vi "Test Modbus.vi"() -> ()   [LabVIEW 2020]
uses:
  <vilib>/NI/Modbus Library/API/Modbus API.lvclass/Modbus API.ctl
  <vilib>/NI/Modbus Library/Transmission Data Unit/Transmission Data Unit.lvclass/Transmission Data Unit.ctl
  <vilib>/NI/Modbus Library/Transmission Data Unit/Write Unit ID.vi
  <vilib>/NI/Modbus Library/API/Read Transmission Data Unit.vi
  <vilib>/NI/Modbus Library/API/Write Transmission Data Unit.vi
  <vilib>/NI/Modbus Library/API/Master/Modbus Master.lvclass
  C:/Program Files (x86)/National Instruments/LabVIEW 2020/vi.lib/NI/Modbus Library/API/Modbus API.lvclass
  <vilib>/NI/Modbus Library/API/Wrapper/Create TCP Master.vi
  <vilib>/NI/Modbus Library/API/Wrapper/API Main.lvlib
panel:
  out "Array 2":dbl[](array[numeric])
  in  "Btn_Set Unit ID":bool
  in  "unit ID":u8
  in  "Array":T1(array[cluster])
  in  "stop":bool
  in  "port (502)":u16=502
  in  "address":string
  in  "Btn_Connect":bool
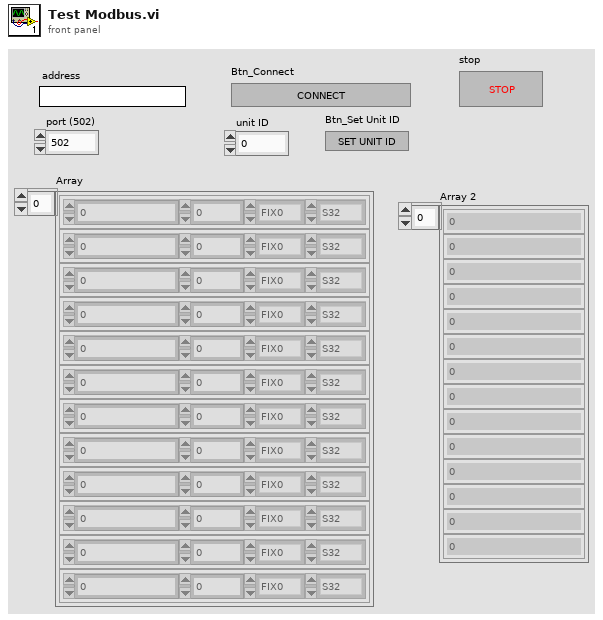
[diagram p1: front panel]
types:
  T1 = cluster{"starting address":u16, "number of inputs":u16, "Data Format":enum16{"FIX0", "FIX1", "FIX2", "FIX3", "FIX4", "FIX5", "FIX6"}, "Data Type":enum16{"S32", "U32"}}[]
  T2 = enum16{"FIX0", "FIX1", "FIX2", "FIX3", "FIX4", "FIX5", "FIX6"}
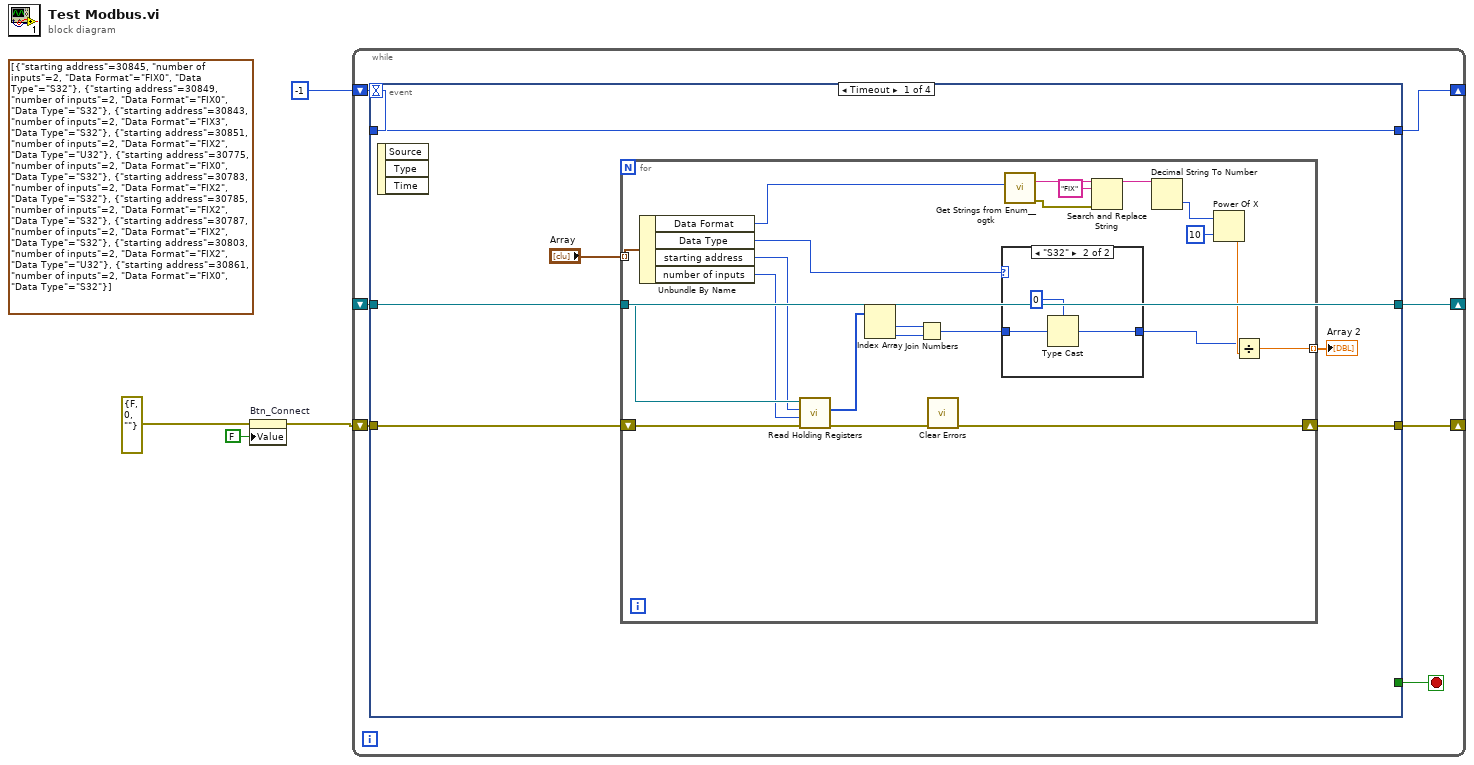
[diagram p0: block diagram]
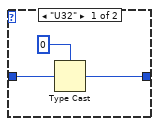
[diagram p2: hidden frame]
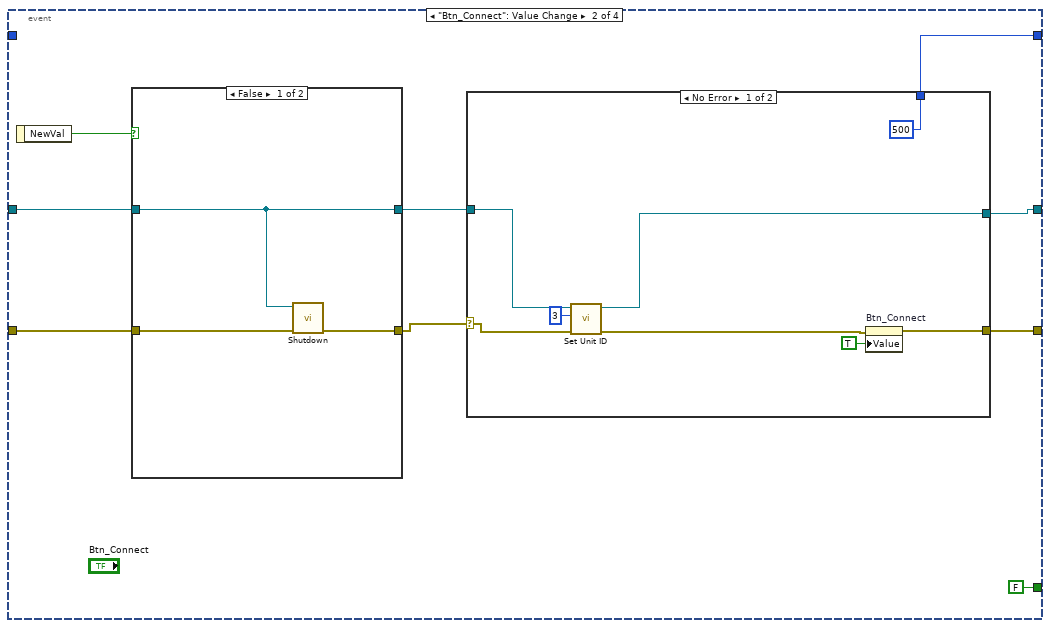
[diagram p3: hidden frame]
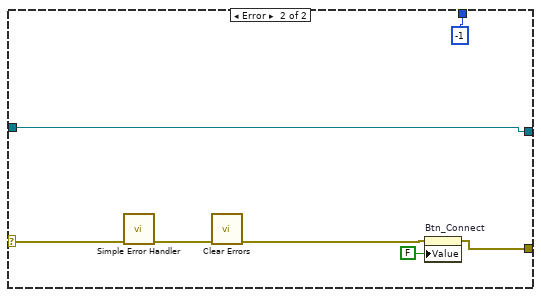
[diagram p4: hidden frame]
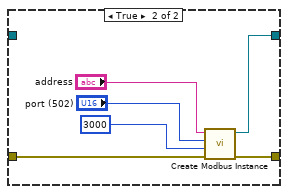
[diagram p5: hidden frame]
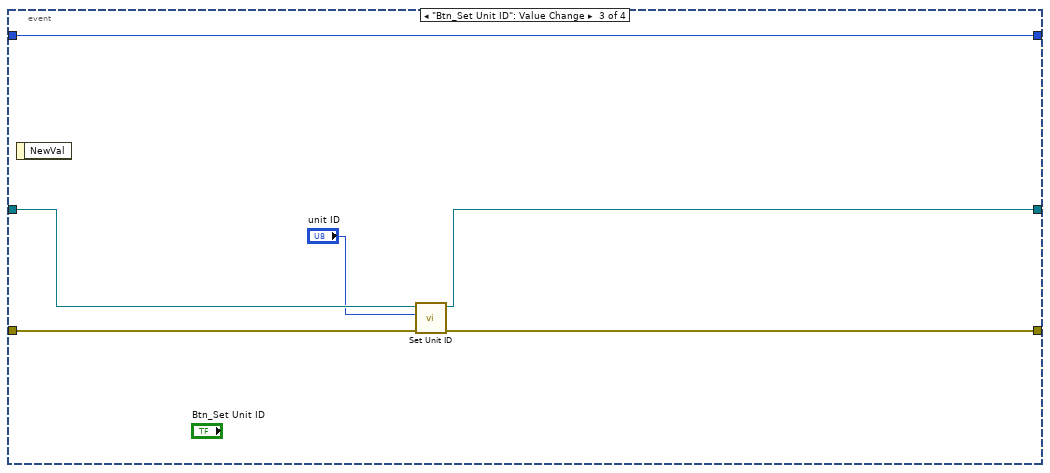
[diagram p6: hidden frame]
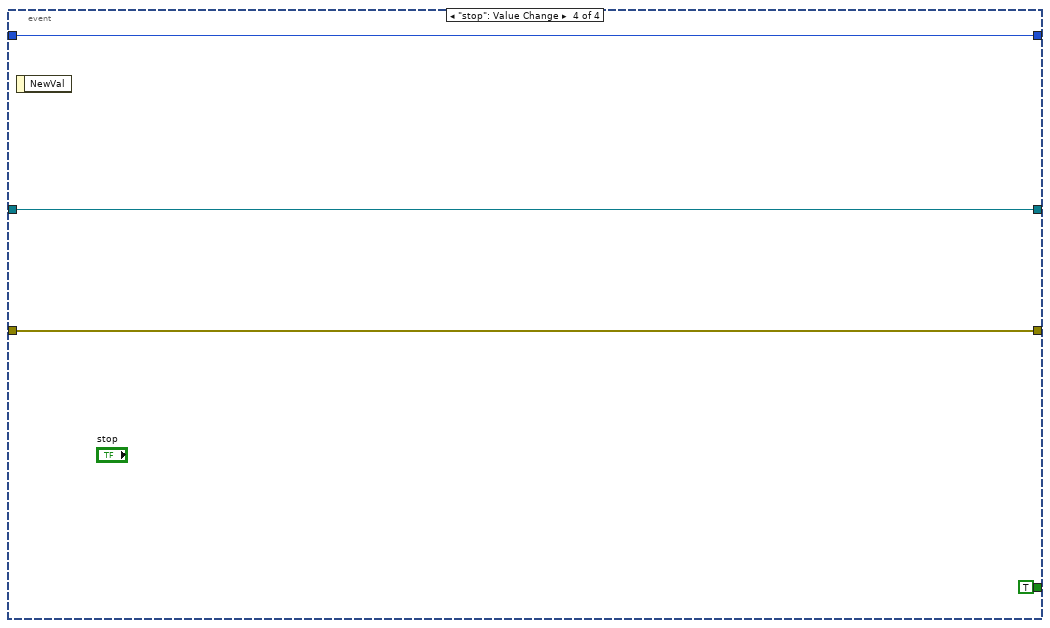
[diagram p7: hidden frame]
diagram:
  (unwired) T1 [{"starting address"=30845, "number of inputs"=2, "Data Format"=enum."FIX0", "Data Type"=enum."S32"}, {"starting address"=30849, "number of inputs"=2, "Data Format"=enum."FIX0", "Data Type"=enum."S32"}, {"starting address"=30843, "number of inputs"=2, "Data Format"=enum."FIX3", "Data Type"=enum."S32"}, {"starting address"=30851, "number of inputs"=2, "Data Format"=enum."FIX2", "Data Type"=enum."U32"}, {"starting address"=30775, "number of inputs"=2, "Data Format"=enum."FIX0", "Data Type"=enum."S32"}, {"starting address"=30783, "number of inputs"=2, "Data Format"=enum."FIX2", "Data Type"=enum."S32"}, {"starting address"=30785, "number of inputs"=2, "Data Format"=enum."FIX2", "Data Type"=enum."S32"}, {"starting address"=30787, "number of inputs"=2, "Data Format"=enum."FIX2", "Data Type"=enum."S32"}, {"starting address"=30803, "number of inputs"=2, "Data Format"=enum."FIX2", "Data Type"=enum."U32"}, {"starting address"=30861, "number of inputs"=2, "Data Format"=enum."FIX0", "Data Type"=enum."S32"}] ("Array")
  n1 = property on="Btn_Connect" class="Bool (strict)"(error in=errorcluster {"status"=FALSE, "code"=0, "source"=""} ("error out"), "Value"=FALSE ("Btn_Connect")) -> (error out=w3:errorcluster)  [unwired: 1 in, 1 out]
  n2 = while {
    shift-right: [w5] -> _
    shift-left: w3 -> [w11]
    shift-right: [w10] -> _
    shift-left: _ -> [w9]
    shift-right: [w6] -> _
    shift-left: -1 -> [w7]
    stop <- w8 stop-if-true
    n3 = event shown="[0] Timeout" {
      selector: _ -> [_ _ _ _]
      dyn-events: _ -> [_ _ _ _]
      timeout: w7 -> [_ _ _ _]
      tunnel: [w15 w50 w83 w87] -> w5
      tunnel: w11 -> [w16 w53 w84 w87]
      tunnel: [w14 w47 w81 w86] -> w10
      tunnel: w9 -> [w14 w52 w82 w86]
      tunnel: [_ FALSE _ TRUE] -> w8
      tunnel: w7 -> [w17 _ w79 w85]
      tunnel: [w17 w49 w79 w85] -> w6
      event Timeout {
        n4 = event-data() -> ()  [unwired: 1 in, 3 out]
        n5 = for {
          tunnel: w14 -> [w37]
          shift-right: [w29] -> w15
          shift-left: w16 -> [w39]
          tunnel: "Array" -> [w36] mode=indexing
          tunnel: [w30] -> w12 mode=indexing
          n6 = Unbundle By Name(w36) -> ("Data Format"=w21:T2, "Data Type"=w20:enum16{"S32", "U32"}, "starting address"=w35:u16, "number of inputs"=w34:u16)
          n7 = call-dynamic "Read Holding Registers.vi"("error in"=w39, "number of inputs"=w34, "starting address"=w35, "Modbus master in"=w37) -> ("error out"=w38:errorcluster, "register values"=w31:u16[])  [unwired: 5 in, 1 out]
          n8 = Index Array(array=w31) -> (element #1=w33:u16, element #2=w32:u16)  [unwired: 2 in]
          n9 = Join Numbers(hi=w33, lo=w32) -> ((hi.lo)=w19:u32)
          n10 = call <vilib>:"Clear Errors.vi"("error in (no error)"=w38) -> ("error out"=w29:errorcluster)  [unwired: 5 in, 1 out]
          n11 = case shown="\"S32\"" w20 {
            tunnel: w19 -> [w42 w45]
            tunnel: [w41 w44] -> w18
            frame "U32" {
              n12 = Type Cast(type=u32 0, x=w42) -> (*(type *) &x=w41:u32)
            }
            frame "S32" {
              n13 = Type Cast(type=0, x=w45) -> (*(type *) &x=w44:i32)
            }
          }
          n14 = call <userlib>:"Get Strings from Enum__ogtk.vi"("Enum"=w21) -> ("error out"=w28:errorcluster, "String Value"=w27:string)  [unwired: 7 in, 2 out]
          n15 = Search and Replace String(input string=w27, search string="FIX", error in=w28) -> (result string=w25:string)  [unwired: 5 in, 3 out]
          n16 = Decimal String To Number(string=w25) -> (number=w24:i32)  [unwired: 2 in, 1 out]
          n17 = Power Of X(1:10 ("x"), 2:w24) -> (0:w22:dbl)
          n18 = Divide(x=w18, y=w22) -> (x/y=w30:dbl)
        }
        "Array 2" <- w12
      }
      event "Btn_Connect": Value Change {
        n19 = event-data() -> ("NewVal"=w54:bool)  [unwired: 1 in]
        n20 = case shown="False" w54 {
          tunnel: w53 -> [w72 w76]
          tunnel: [w71 w74] -> w48
          tunnel: w52 -> [w71 _]
          tunnel: [w70 w73] -> w46
          frame False {
            n21 = call-dynamic "Shutdown.vi"("error in"=w72, "Modbus master in"=w71) -> ("error out"=w70:errorcluster)  [unwired: 9 in]
          }
          frame True {
            n22 = call-poly <vilib>:"Create Modbus Instance.vi"("error in"=w76, "connect timeout ms"=3000, "port (502)"="port (502)", "address"="address") -> ("error out"=w73:errorcluster, "TCP master instance"=w74:refnum<class "Modbus Master.lvclass">)  [unwired: 6 in]
          }
        }
        n23 = case shown="No Error" w46 {
          selector: w46 -> [w55 w67]
          tunnel: [w62 w68] -> w50
          tunnel: [500 -1] -> w49
          tunnel: w48 -> [w60 w64]
          tunnel: [w59 w64] -> w47
          frame No Error {
            n24 = call <vilib>:"Set Unit ID.vi"("error in"=w55, "unit ID"=u8 3, "Modbus master in"=w60) -> ("error out"=w57:errorcluster, "Modbus master out"=w59:refnum<class "Modbus Master.lvclass">)  [unwired: 7 in]
            n25 = property on="Btn_Connect" class="Bool (strict)"(error in=w57, "Value"=TRUE ("Btn_Connect")) -> (error out=w62:errorcluster)  [unwired: 1 in, 1 out]
          }
          frame Error {
            n26 = call <vilib>:"Simple Error Handler.vi"("error in (no error)"=w67) -> ("error out"=w66:errorcluster)  [unwired: 4 in, 4 out]
            n27 = call <vilib>:"Clear Errors.vi"("error in (no error)"=w66) -> ("error out"=w65:errorcluster)  [unwired: 5 in, 1 out]
            n28 = property on="Btn_Connect" class="Bool (strict)"(error in=w65, "Value"=FALSE ("Btn_Connect")) -> (error out=w68:errorcluster)  [unwired: 1 in, 1 out]
          }
        }
      }
      event "Btn_Set Unit ID": Value Change {
        n29 = event-data() -> ()  [unwired: 1 in, 1 out]
        n30 = call <vilib>:"Set Unit ID.vi"("error in"=w84, "unit ID"="unit ID", "Modbus master in"=w82) -> ("error out"=w83:errorcluster, "Modbus master out"=w81:refnum<class "Modbus Master.lvclass">)  [unwired: 7 in]
      }
      event "stop": Value Change {
        n31 = event-data() -> ()  [unwired: 1 in, 1 out]
      }
    }
  }
